vi "Speaker ring to Text.vi"(1 "Speaker":T1) -> (0 "Text":string)   [LabVIEW 2020]
uses:
  Speaker ring.ctl
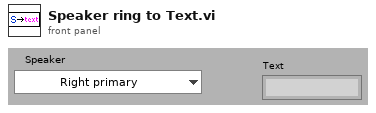
[diagram p1: front panel]
types:
  T1 = typedef "Speaker ring.ctl" = enum16{"Right primary", "Right secondary", "Left primary", "Left secondary"}
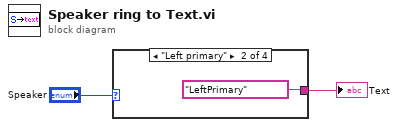
[diagram p0: block diagram]
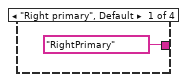
[diagram p2: hidden frame]
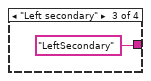
[diagram p3: hidden frame]
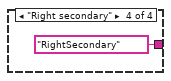
[diagram p4: hidden frame]
diagram:
  n1 = case shown="\"Left primary\"" "Speaker" {
    tunnel: ["RightPrimary" "LeftPrimary" "LeftSecondary" "RightSecondary"] -> w1
    frame "Right primary", Default {
    }
    frame "Left primary" {
    }
    frame "Left secondary" {
    }
    frame "Right secondary" {
    }
  }
  "Text" <- w1
